vi "Final_Project_Software_Abhishek_Barla.vi"(10 "Type of Image":enum16{"JPEG Image", "BMP Image", "PNG Image"}(ring) caption="Select the Type of Image", 11 "?":path) -> ()   [LabVIEW 2015]
uses:
  <vilib>/measure/NI_MABase.lvlib
  <vilib>/Analysis/NI_AALBase.lvlib
panel:
  out "resulting string":string
  out "Decoded R Channel with Text Buried":string
  out "Image with Text Buried":picture
  out "R Channel Array":u8[](array[numeric])
  out "R Channel With Intelligence":u8[](array[numeric])
  out "Buried Text Array":u8[](array[numeric])
  out "Burried Text Array Indexed":u8[](array[numeric])
  out "Converted String":string
  in  "Binary or HEX":bool caption="String Conversion"
  out "String from the Text File":string
  in  "?":path
  out "Filtered Image":picture
  in  "Type of Filter":T1(ring) caption="Select the Type of Filter to be Applied"
  out "Combined Noisy Image":picture
  out "Noisy Image - B Channel":picture
  out "Noisy Image - G Channel":picture
  out "Noisy Image - R Channel":picture
  in  "Type of Noise":T2(ring) caption="Select Type of Noise for G Channel"
  in  "Type of Noise":T2(ring) caption="Select Type of Noise for B Channel"
  in  "Type of Noise":T3(ring) caption="Select Type of Noise for R Channel"
  out "Original Image":picture
  # "Virtual Instrumentation Lab - Spring 2015 Final Project - Abhishek Barla"
  # "Please Select a 200x200 Picture"
  # "Select the Text File to Read"
  # "Binary"
  # "Hexadecimal"
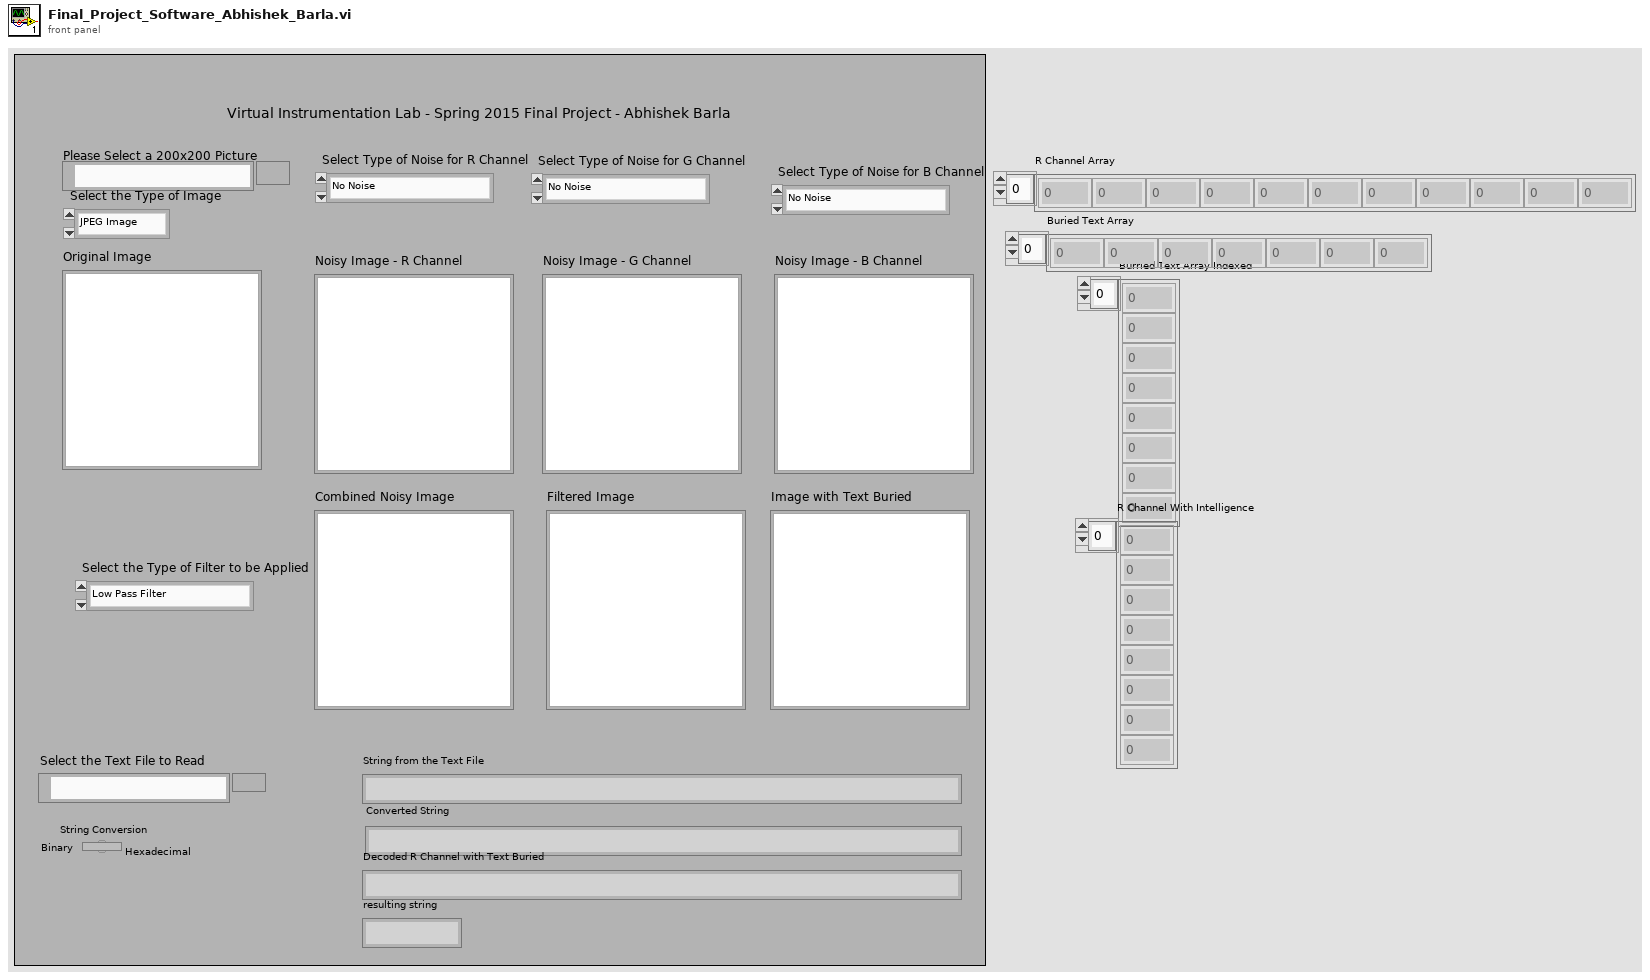
[diagram p1: front panel]
types:
  T1 = enum16{"Low Pass Filter", "High Pass Filter", "Band Pass Filter", "Band Stop Filter", "Median Filter"}
  T2 = enum16{"No Noise", "Gaussian White Noise", "Uniform White Noise", "Periodic Random Noise"}
  T3 = enum16{"No Noise", "Gaussian White Noise", "Uniform White Noise", "Peridoic Random Noise"}
  T4 = typedef "imagedata.ctl" = cluster{"image type":i32, "image depth":i32, "image":u8[], "mask":u8[], "colors":u32[], "Rectangle":cluster{"left":i16, "top":i16, "right":i16, "bottom":i16}}
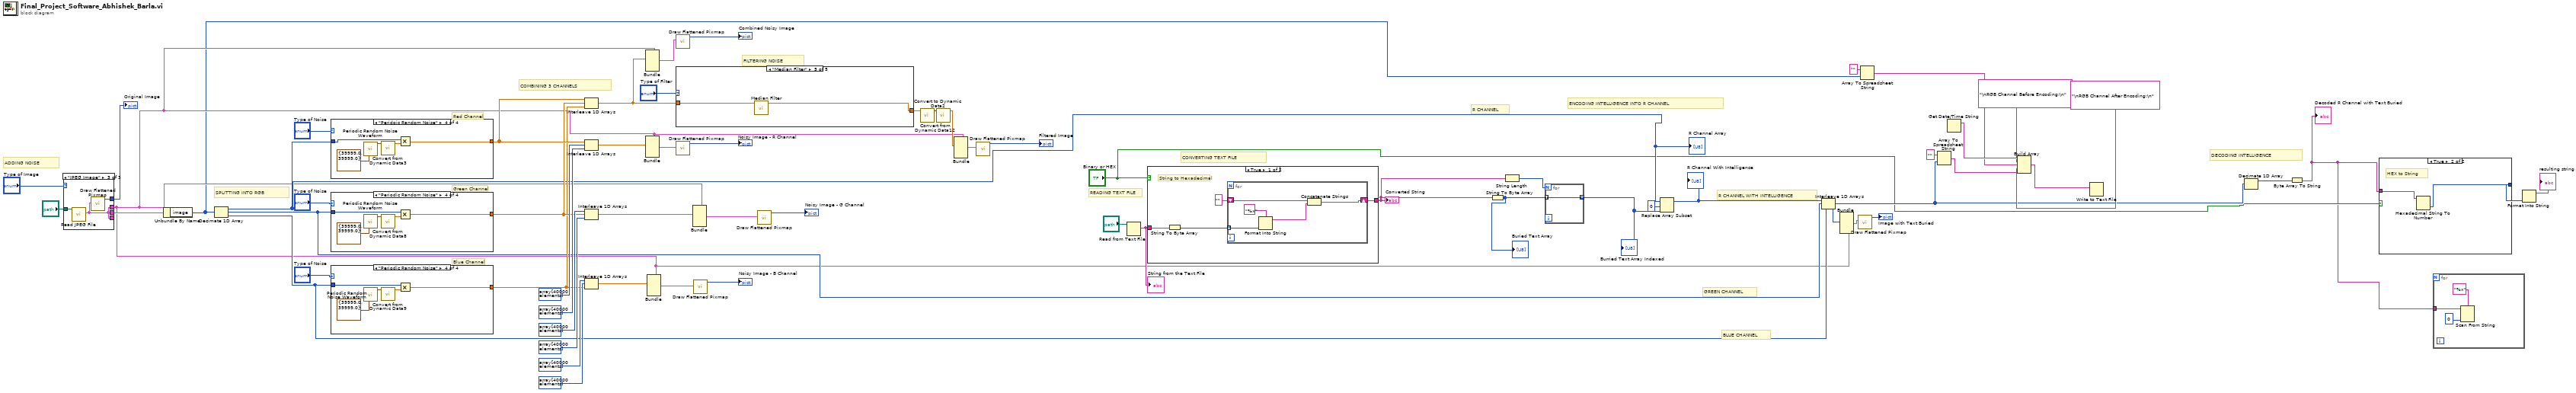
[diagram p0: block diagram]
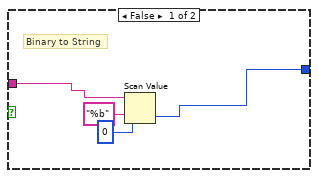
[diagram p2: hidden frame]
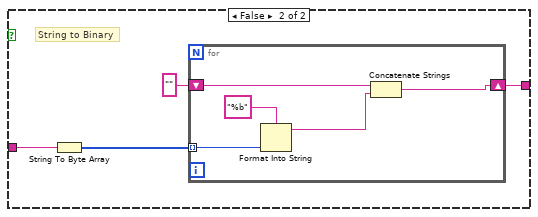
[diagram p3: hidden frame]
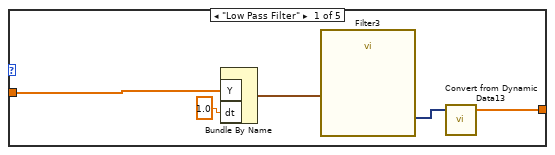
[diagram p4: hidden frame]
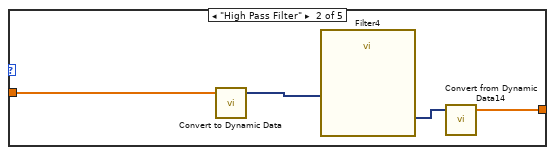
[diagram p5: hidden frame]
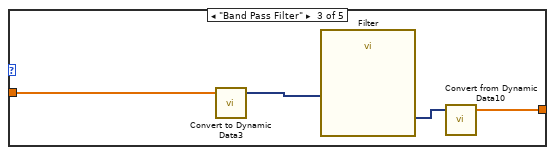
[diagram p6: hidden frame]
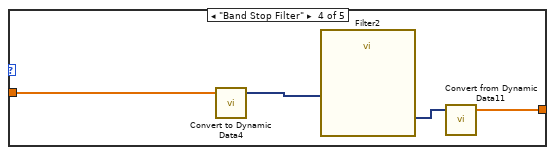
[diagram p7: hidden frame]
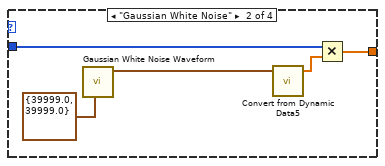
[diagram p9: hidden frame]
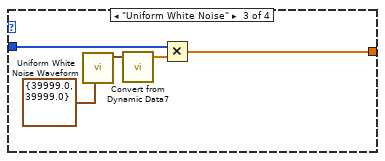
[diagram p10: hidden frame]
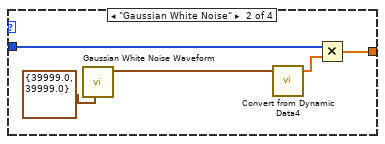
[diagram p12: hidden frame]
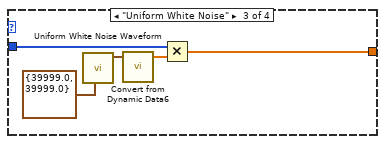
[diagram p13: hidden frame]
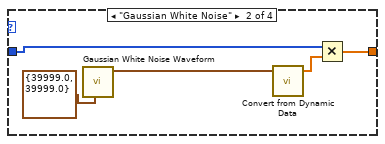
[diagram p15: hidden frame]
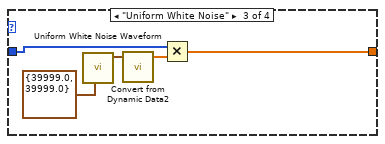
[diagram p16: hidden frame]
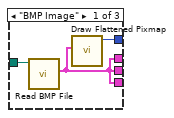
[diagram p17: hidden frame]
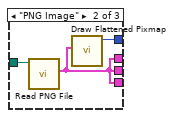
[diagram p18: hidden frame]
diagram:
  # "DECODING INTELLIGENCE"
  # "BLUE CHANNEL"
  # "GREEN CHANNEL"
  # "R CHANNEL WITH INTELLIGENCE"
  # "R CHANNEL"
  # "ENCODING INTELLIGENCE INTO R CHANNEL"
  # "CONVERTING TEXT FILE"
  # "READING TEXT FILE"
  # "FILTERING NOISE"
  # "COMBINING 3 CHANNELS"
  # "SPLITTING INTO RGB"
  # "ADDING NOISE"
  # "Blue Channel"
  # "Green Channel"
  # "Red Channel"
  n1 = case shown="\"JPEG Image\"" "Type of Image" {
    tunnel: "?" -> [w66 w69 w72]
    tunnel: [w65 w68 w71] -> w61
    tunnel: [w64 w67 w70] -> w60
    tunnel: [w64 w67 w70] -> _
    tunnel: [w64 w67 w70] -> w17
    frame "BMP Image" {
      n2 = call <vilib>:"Read BMP File.vi"("path to BMP file"=w66) -> ("image data"=w64:T4)  [unwired: 8 in, 2 out]
      n3 = call <vilib>:"Draw Flattened Pixmap.vi"("image data"=w64) -> ("new picture"=w65:picture)  [unwired: 8 in]
    }
    frame "PNG Image" {
      n4 = call <vilib>:"Read PNG File.vi"("path to PNG file"=w69) -> ("image data"=w67:T4)  [unwired: 8 in, 2 out]
      n5 = call <vilib>:"Draw Flattened Pixmap.vi"("image data"=w67) -> ("new picture"=w68:picture)  [unwired: 8 in]
    }
    frame "JPEG Image" {
      n6 = call <vilib>:"Read JPEG File.vi"("path to JPEG file"=w72) -> ("image data"=w70:T4)  [unwired: 8 in, 2 out]
      n7 = call <vilib>:"Draw Flattened Pixmap.vi"("image data"=w70) -> ("new picture"=w71:picture)  [unwired: 8 in]
    }
  }
  "Original Image" <- w61
  n8 = Unbundle By Name "Unbundle By Name"(w60) -> ("image"=w11:u8[])
  n9 = Decimate 1D Array "Decimate 1D Array"(w11) -> (w23:u8[], w21:u8[], w20:u8[])
  "R Channel Array" <- w23
  n10 = case shown="\"Peridoic Random Noise\"" "Type of Noise" {
    tunnel: w23 -> [w73 w77 w83 w85]
    tunnel: [w73 w78 w80 w87] -> w42
    frame "No Noise", Default {
    }
    frame "Gaussian White Noise" {
      n11 = call <vilib>:"Gaussian White Noise Waveform.vi"("sampling info"=cluster{"Fs":dbl, "#s":dbl} {"Fs"=39999.0, "#s"=39999.0}) -> ("signal out"=w76:waveform(dbl))  [unwired: 9 in, 1 out]
      n12 = call "Convert from Dynamic Data"("Dynamic Data Type"=w76) -> ("Array"=w75:dbl[])  [unwired: 3 in]
      n13 = Multiply(x=w77, y=w75) -> (x*y=w78:dbl[])
    }
    frame "Uniform White Noise" {
      n14 = call <vilib>:"Uniform White Noise Waveform.vi"("sampling info"=cluster{"Fs":dbl, "#s":dbl} {"Fs"=39999.0, "#s"=39999.0}) -> ("signal out"=w82:waveform(dbl))  [unwired: 9 in, 1 out]
      n15 = call "Convert from Dynamic Data2"("Dynamic Data Type"=w82) -> ("Array"=w81:dbl[])  [unwired: 3 in]
      n16 = Multiply(x=w83, y=w81) -> (x*y=w80:dbl[])
    }
    frame "Peridoic Random Noise" {
      n17 = call <vilib>:"Periodic Random Noise Waveform.vi"("sampling info"=cluster{"Fs":dbl, "#s":dbl} {"Fs"=39999.0, "#s"=39999.0}) -> ("signal out"=w88:waveform(dbl))  [unwired: 9 in, 1 out]
      n18 = call "Convert from Dynamic Data3"("Dynamic Data Type"=w88) -> ("Array"=w86:dbl[])  [unwired: 3 in]
      n19 = Multiply(x=w85, y=w86) -> (x*y=w87:dbl[])
    }
  }
  n20 = case shown="\"Periodic Random Noise\"" "Type of Noise" {
    tunnel: w21 -> [w89 w91 w97 w102]
    tunnel: [w89 w92 w96 w101] -> w41
    frame "No Noise", Default {
    }
    frame "Gaussian White Noise" {
      n21 = call <vilib>:"Gaussian White Noise Waveform.vi"("sampling info"=cluster{"Fs":dbl, "#s":dbl} {"Fs"=39999.0, "#s"=39999.0}) -> ("signal out"=w94:waveform(dbl))  [unwired: 9 in, 1 out]
      n22 = call "Convert from Dynamic Data4"("Dynamic Data Type"=w94) -> ("Array"=w93:dbl[])  [unwired: 3 in]
      n23 = Multiply(x=w91, y=w93) -> (x*y=w92:dbl[])
    }
    frame "Uniform White Noise" {
      n24 = call <vilib>:"Uniform White Noise Waveform.vi"("sampling info"=cluster{"Fs":dbl, "#s":dbl} {"Fs"=39999.0, "#s"=39999.0}) -> ("signal out"=w99:waveform(dbl))  [unwired: 9 in, 1 out]
      n25 = call "Convert from Dynamic Data6"("Dynamic Data Type"=w99) -> ("Array"=w98:dbl[])  [unwired: 3 in]
      n26 = Multiply(x=w97, y=w98) -> (x*y=w96:dbl[])
    }
    frame "Periodic Random Noise" {
      n27 = call <vilib>:"Periodic Random Noise Waveform.vi"("sampling info"=cluster{"Fs":dbl, "#s":dbl} {"Fs"=39999.0, "#s"=39999.0}) -> ("signal out"=w104:waveform(dbl))  [unwired: 9 in, 1 out]
      n28 = call "Convert from Dynamic Data8"("Dynamic Data Type"=w104) -> ("Array"=w103:dbl[])  [unwired: 3 in]
      n29 = Multiply(x=w102, y=w103) -> (x*y=w101:dbl[])
    }
  }
  n30 = case shown="\"Periodic Random Noise\"" "Type of Noise" {
    tunnel: w20 -> [w105 w108 w113 w118]
    tunnel: [w105 w107 w112 w117] -> w40
    frame "No Noise", Default {
    }
    frame "Gaussian White Noise" {
      n31 = call <vilib>:"Gaussian White Noise Waveform.vi"("sampling info"=cluster{"Fs":dbl, "#s":dbl} {"Fs"=39999.0, "#s"=39999.0}) -> ("signal out"=w110:waveform(dbl))  [unwired: 9 in, 1 out]
      n32 = call "Convert from Dynamic Data5"("Dynamic Data Type"=w110) -> ("Array"=w109:dbl[])  [unwired: 3 in]
      n33 = Multiply(x=w108, y=w109) -> (x*y=w107:dbl[])
    }
    frame "Uniform White Noise" {
      n34 = call <vilib>:"Uniform White Noise Waveform.vi"("sampling info"=cluster{"Fs":dbl, "#s":dbl} {"Fs"=39999.0, "#s"=39999.0}) -> ("signal out"=w115:waveform(dbl))  [unwired: 9 in, 1 out]
      n35 = call "Convert from Dynamic Data7"("Dynamic Data Type"=w115) -> ("Array"=w114:dbl[])  [unwired: 3 in]
      n36 = Multiply(x=w113, y=w114) -> (x*y=w112:dbl[])
    }
    frame "Periodic Random Noise" {
      n37 = call <vilib>:"Periodic Random Noise Waveform.vi"("sampling info"=cluster{"Fs":dbl, "#s":dbl} {"Fs"=39999.0, "#s"=39999.0}) -> ("signal out"=w120:waveform(dbl))  [unwired: 9 in, 1 out]
      n38 = call "Convert from Dynamic Data9"("Dynamic Data Type"=w120) -> ("Array"=w119:dbl[])  [unwired: 3 in]
      n39 = Multiply(x=w118, y=w119) -> (x*y=w117:dbl[])
    }
  }
  n40 = Interleave 1D Arrays "Interleave 1D Arrays"(w42, w41, w40) -> (w36:dbl[])
  n41 = Interleave 1D Arrays "Interleave 1D Arrays"(w42, u8[] array[40000 elements] ("array"), u8[] array[40000 elements] ("array")) -> (w30:dbl[])
  n42 = Interleave 1D Arrays "Interleave 1D Arrays"(u8[] array[40000 elements] ("array"), w41, u8[] array[40000 elements] ("array")) -> (w43:dbl[])
  n43 = Interleave 1D Arrays "Interleave 1D Arrays"(u8[] array[40000 elements] ("array"), u8[] array[40000 elements] ("array"), w40) -> (w48:dbl[])
  n44 = Bundle "Bundle"(cluster=w17, "image"=w36) -> (w38:T4)  [unwired: 5 in]
  n45 = Bundle "Bundle"(cluster=w17, "image"=w30) -> (w57:T4)  [unwired: 5 in]
  n46 = Bundle(cluster=w17, "image"=w48) -> (w53:T4)  [unwired: 5 in]
  n47 = call <vilib>:"Draw Flattened Pixmap.vi"("image data"=w38) -> ("new picture"=→"Combined Noisy Image":picture)  [unwired: 8 in]
  n48 = case shown="\"Median Filter\"" "Type of Filter" {
    tunnel: w36 -> [w123 w129 w133 w137 w139]
    tunnel: [w121 w126 w130 w134 w138] -> w32
    frame "Low Pass Filter" {
      n49 = Bundle By Name("Y"=w123, "dt"=1.0) -> (w124:waveform(dbl))  [unwired: 1 in]
      n50 = call "Filter3"("Signal"=w124) -> ("Filtered Signal"=w122:dynamicdata)  [unwired: 9 in, 1 out]
      n51 = call "Convert from Dynamic Data13"("Dynamic Data Type"=w122) -> ("Array"=w121:dbl[])  [unwired: 3 in]
    }
    frame "High Pass Filter" {
      n52 = call "Convert to Dynamic Data"("Array"=w129) -> ("Dynamic Data Type"=w128:dynamicdata)  [unwired: 3 in]
      n53 = call "Filter4"("Signal"=w128) -> ("Filtered Signal"=w127:dynamicdata)  [unwired: 9 in, 1 out]
      n54 = call "Convert from Dynamic Data14"("Dynamic Data Type"=w127) -> ("Array"=w126:dbl[])  [unwired: 3 in]
    }
    frame "Band Pass Filter" {
      n55 = call "Convert to Dynamic Data3"("Array"=w133) -> ("Dynamic Data Type"=w132:dynamicdata)  [unwired: 3 in]
      n56 = call "Filter"("Signal"=w132) -> ("Filtered Signal"=w131:dynamicdata)  [unwired: 9 in, 1 out]
      n57 = call "Convert from Dynamic Data10"("Dynamic Data Type"=w131) -> ("Array"=w130:dbl[])  [unwired: 3 in]
    }
    frame "Band Stop Filter" {
      n58 = call "Convert to Dynamic Data4"("Array"=w137) -> ("Dynamic Data Type"=w136:dynamicdata)  [unwired: 3 in]
      n59 = call "Filter2"("Signal"=w136) -> ("Filtered Signal"=w135:dynamicdata)  [unwired: 9 in, 1 out]
      n60 = call "Convert from Dynamic Data11"("Dynamic Data Type"=w135) -> ("Array"=w134:dbl[])  [unwired: 3 in]
    }
    frame "Median Filter" {
      n61 = call <vilib>:"Median Filter.vi"("X"=w139) -> ("Filtered X"=w138:dbl[])  [unwired: 9 in, 1 out]
    }
  }
  n62 = call <vilib>:"Draw Flattened Pixmap.vi"("image data"=w57) -> ("new picture"=→"Noisy Image - R Channel":picture)  [unwired: 8 in]
  n63 = Bundle(cluster=w17, "image"=w43) -> (w55:T4)  [unwired: 5 in]
  n64 = call <vilib>:"Draw Flattened Pixmap.vi"("image data"=w53) -> ("new picture"=→"Noisy Image - B Channel":picture)  [unwired: 8 in]
  n65 = call <vilib>:"Draw Flattened Pixmap.vi"("image data"=w55) -> ("new picture"=→"Noisy Image - G Channel":picture)  [unwired: 8 in]
  n66 = call "Convert to Dynamic Data2"("Array"=w32) -> ("Dynamic Data Type"=w31:dynamicdata)  [unwired: 3 in]
  n67 = call "Convert from Dynamic Data12"("Dynamic Data Type"=w31) -> ("Array"=w34:dbl[])  [unwired: 3 in]
  n68 = Bundle "Bundle"(cluster=w17, "image"=w34) -> (w33:T4)  [unwired: 5 in]
  n69 = call <vilib>:"Draw Flattened Pixmap.vi"("image data"=w33) -> ("new picture"=→"Filtered Image":picture)  [unwired: 8 in]
  n70 = Read from Text File(file (use dialog)="?") -> (text=w28:string)  [unwired: 3 in, 3 out]
  "String from the Text File" <- w28
  n71 = case shown="True" "Binary or HEX" {
    tunnel: w28 -> [w143 w152]
    tunnel: [w140 w149] -> w27
    frame True {
      # "String to Hexadecimal"
      n72 = String To Byte Array(string=w143) -> (unsigned byte array=w142:u8[])
      n73 = for {
        tunnel: w142 -> [w146] mode=indexing
        shift-right: [w148] -> w140
        shift-left: "" -> [w147]
        n74 = Format Into String "Format Into String"(format string="%x", w146) -> (resulting string=w145:string)  [unwired: 2 in, 1 out]
        n75 = Concatenate Strings "Concatenate Strings"(w147, w145) -> (w148:string)
      }
    }
    frame False {
      # "String to Binary"
      n76 = String To Byte Array(string=w152) -> (unsigned byte array=w151:u8[])
      n77 = for {
        tunnel: w151 -> [w156] mode=indexing
        shift-right: [w157] -> w149
        shift-left: "" -> [w153]
        n78 = Format Into String "Format Into String"(format string="%b", w156) -> (resulting string=w155:string)  [unwired: 2 in, 1 out]
        n79 = Concatenate Strings "Concatenate Strings"(w153, w155) -> (w157:string)
      }
    }
  }
  "Converted String" <- w27
  n80 = String To Byte Array(string=w27) -> (unsigned byte array=w24:u8[])
  "Buried Text Array" <- w24
  n81 = String Length(string=w27) -> (length=w7:i32)
  n82 = for {
    N: w7 -> [_]
    tunnel: [w158] -> w26 mode=indexing
    tunnel: w24 -> [w158] mode=indexing
  }
  "Burried Text Array Indexed" <- w26
  n83 = Replace Array Subset "Replace Array Subset"(array=w23, new element=w26, index=0) -> (w22:u8[])
  "R Channel With Intelligence" <- w22
  n84 = Interleave 1D Arrays "Interleave 1D Arrays"(w22, w21, w20) -> (w5:u8[])
  n85 = Bundle(cluster=w17, "image"=w5) -> (w18:T4)  [unwired: 5 in]
  n86 = call <vilib>:"Draw Flattened Pixmap.vi"("image data"=w18) -> ("new picture"=→"Image with Text Buried":picture)  [unwired: 8 in]
  n87 = Array To Spreadsheet String(array=w11, 3:"" ("format string")) -> (spreadsheet string=w10:string)  [unwired: 1 in]
  n88 = Array To Spreadsheet String(array=w5, 3:"" ("format string")) -> (spreadsheet string=w8:string)  [unwired: 1 in]
  n89 = Get Date/Time String() -> (date string=w14:string)  [unwired: 3 in, 1 out]
  n90 = Build Array "Build Array"(w14, "\nRGB Channel Before Encoding:\n" ("element"), w10, "\nRGB Channel After Encoding:\n" ("element"), w8) -> (w15:string[])
  n91 = Write to Text File(text=w15) -> ()  [unwired: 3 in, 3 out]
  n92 = Decimate 1D Array "Decimate 1D Array"(w5) -> (w6:u8[])  [unwired: 2 out]
  n93 = Byte Array To String(unsigned byte array=w6) -> (string=w1:string)
  "Decoded R Channel with Text Buried" <- w1
  n94 = case shown="True" "Binary or HEX" {
    tunnel: w1 -> [w160 w163]
    tunnel: [w159 w164] -> w2
    frame False {
      # "Binary to String"
      n95 = Scan Value(string=w160, format string="%b", default (0 dbl)=u32 0) -> (value=w159:u32)  [unwired: 1 out]
    }
    frame True {
      # "HEX to String"
      n96 = Hexadecimal String To Number(string=w163) -> (number=w164:u32)  [unwired: 2 in, 1 out]
    }
  }
  n97 = for {
    tunnel: w1 -> [w167]
    n98 = Scan From String "Scan From String"(format string="%x", input string=w167, default 1=0) -> ()  [unwired: 3 in, 3 out]
  }
  n99 = Format Into String "Format Into String"(w2) -> (resulting string=→"resulting string":string)  [unwired: 3 in, 1 out]
